vi "_PC_Pub_VIAllControlDisable.vi"(8 "error in (no error)":errorcluster, 10 "Disabled":T1(ring), 11 "VI reference in":refnum<vi>) -> (0 "error out":errorcluster, 3 "VI reference out":refnum<vi>)   [LabVIEW 2016]
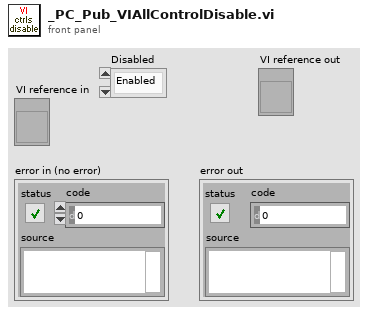
[diagram p1: front panel]
types:
  T1 = enum8{"Enabled", "Disabled", "Disabled and Grayed Out"}
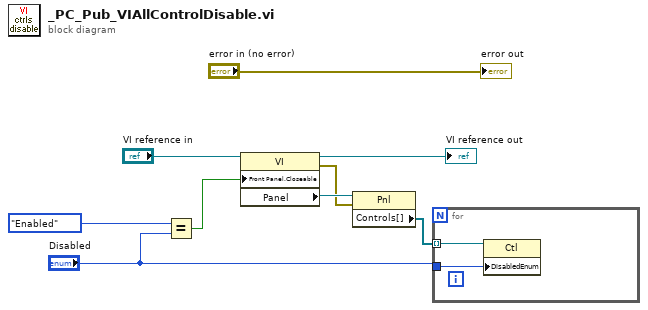
[diagram p0: block diagram]
diagram:
  n1 = Equal?(x=T1."Enabled", y="Disabled") -> (x = y?=w3:bool)
  n2 = property class="VI"(reference="VI reference in", "Front Panel.Closeable"=w3) -> (reference out=→"VI reference out":refnum<vi>, error out=w6:errorcluster, "Panel"=w8:refnum<vi>)  [unwired: 1 in]
  n3 = property class="Pnl"(reference=w8, error in=w6) -> ("Controls[]"=w9:refnum<vi>[])  [unwired: 2 out]
  n4 = for {
    tunnel: w9 -> [w11] mode=indexing
    tunnel: "Disabled" -> [w10]
    n5 = property class="Ctl"(reference=w11, "DisabledEnum"=w10) -> ()  [unwired: 1 in, 2 out]
  }
  "error out" <- "error in (no error)"
